vi "Resistance Measuring 2182A.vi"() -> ()   [LabVIEW 2022 SP3]
uses:
  <instrlib>/Keithley 2182/Keithley 2182.lvlib
panel:
  out "Measurements":dbl[][](array[numeric])
  in  "Integration Rate (5)":dbl=5.0
  in  "Range Value (12)":dbl=12.0
  in  "Voltage Resolution (8)":i32=8
  in  "Measurement (0: Voltage Channel 1)":i32(ring) items=["Voltage Channel 1", "Voltage Channel 2", "Temperature Channel 1", "Temperature Channel 2"]
  in  "Number of Measurements":u32=5
  in  "VISA NanoVoltmeter":refnum<visa-resource-name>
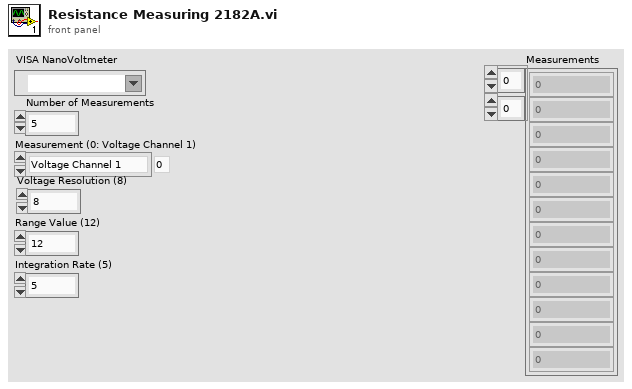
[diagram p1: front panel]
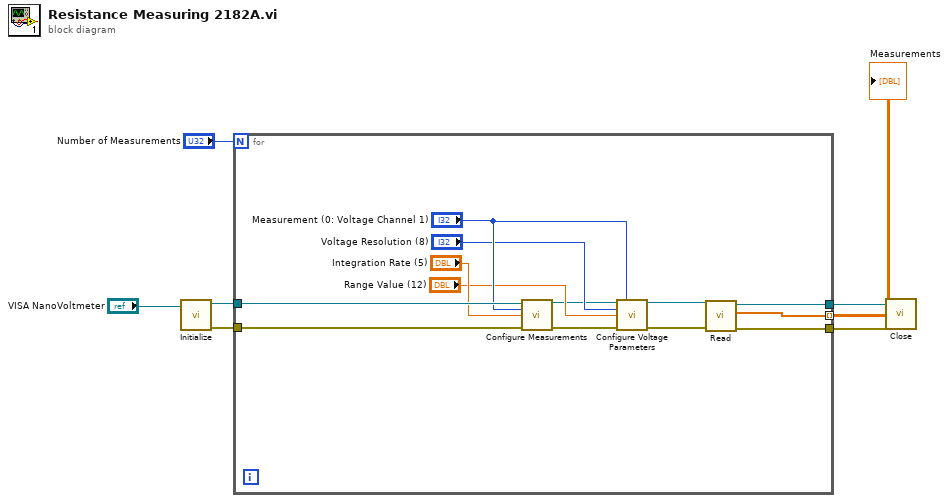
[diagram p0: block diagram]
diagram:
  n1 = call <instrlib>:"Initialize.vi"("VISA resource name"="VISA NanoVoltmeter") -> ("error out"=w4:errorcluster, "VISA resource name out"=w5:refnum<visa-resource-name>)  [unwired: 9 in]
  n2 = for {
    N: "Number of Measurements" -> [_]
    tunnel: w5 -> [w20]
    tunnel: w4 -> [w19]
    tunnel: [w11] -> w3
    tunnel: [w10] -> w2
    tunnel: [w9] -> w1 mode=indexing
    n3 = call <instrlib>:"Configure Measurements.vi"("VISA resource name"=w20, "Measurement (0: Voltage Channel 1)"="Measurement (0: Voltage Channel 1)", "Integration Rate (5)"="Integration Rate (5)", "error in (no error)"=w19) -> ("VISA resource name out"=w8:refnum<visa-resource-name>, "error out"=w12:errorcluster)  [unwired: 10 in]
    n4 = call <instrlib>:"Configure Voltage Parameters.vi"("VISA resource name"=w8, "Measurement (1: Voltage Channel 1)"="Measurement (0: Voltage Channel 1)", "Voltage Resolution (8)"="Voltage Resolution (8)", "Range Value (12)"="Range Value (12)", "error in (no error)"=w12) -> ("VISA resource name out"=w14:refnum<visa-resource-name>, "error out"=w13:errorcluster)  [unwired: 9 in]
    n5 = call <instrlib>:"Read.vi"("error in (no error)"=w13, "VISA resource name"=w14) -> ("error out"=w10:errorcluster, "Measurements"=w9:dbl[], "VISA resource name out"=w11:refnum<visa-resource-name>)  [unwired: 6 in, 1 out]
  }
  "Measurements" <- w1
  n6 = call <instrlib>:"Close.vi"("error in (no error)"=w2, "VISA resource name"=w3) -> ()  [unwired: 9 in, 1 out]
